vi "Read Single Raw Waveform.vi"(4 "Arm trigger":bool, 6 "Custom Source ID":string, 8 "error in (no error)":errorcluster, 9 "Timeout (10000 ms)":u32=10000, 10 "Source (0: Channel 1)":u16(ring) items=["Channel 1", "Channel 2", "Channel 3", "Channel 4", "Memory 1", "Memory 2", "Memory 3", "Memory 4", "Function 1", "Function 2", "Function 3", "Function 4", "Function 5", "Function 6", "Function 7", "Function 8", "Other"], 11 "VISA resource name":refnum<visa-resource-name>) -> (0 "error out":errorcluster, 2 "Waveform Data":waveform(i16)(graph), 3 "VISA resource name out":refnum<visa-resource-name>, 5 "Vertical offset":sgl, 7 "Vertical gain":sgl)   [LabVIEW 2018, in "LeCroy Wave Series.lvlib"]
doc: "Initiates an acquisition on all channels that you enabled with the <B>Configure Channel</B> VI. The VI waits for the acquisition to complete and returns the waveform for the Source channel you specified. If the oscilloscope did not complete the acquisition within the time period you specify with the Timeout parameter, the VI returns a time out error. A common cause for a timeout error is the acquisition was not triggered. For example, the trigger level is out of range of the waveform.\n\nCall the <B>Fetch Waveform</B> VI to obtain the waveforms for each of the remaining enabled Source channels without initiating another acquisition.\n\nNote: If your instrument does not support auto compensation for probe attenuation, you may need to adjust the scaling of the Waveform Data accordingly. This is handled automatically in the <B>Configure Channel</B> VI or can be done manually by multiplying the Waveform Data by the probe attenuation."
uses:
  LeCroy Wave Series.lvlib
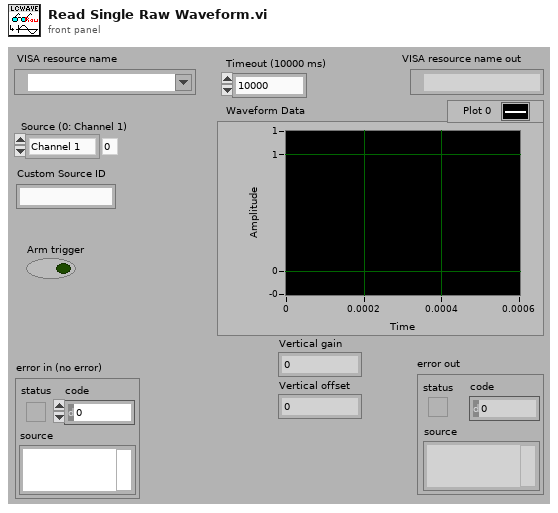
[diagram p1: front panel]
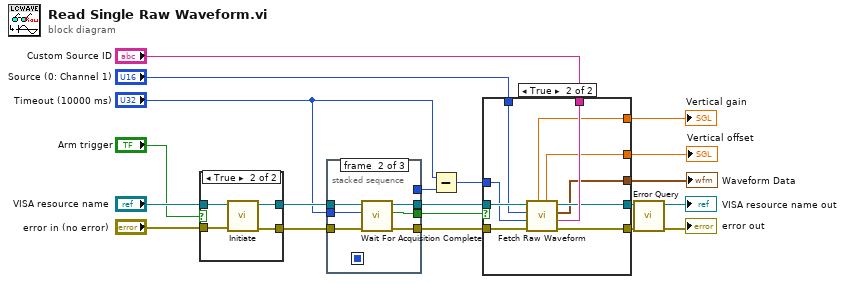
[diagram p0: block diagram]
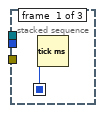
[diagram p4: hidden frame]
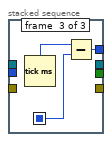
[diagram p5: hidden frame]
diagram:
  n1 = case shown="True" "Arm trigger" {
    tunnel: "VISA resource name" -> [w22 w26]
    tunnel: "error in (no error)" -> [w21 w25]
    tunnel: [w22 w24] -> w12
    tunnel: [w21 w23] -> w11
    frame False {
    }
    frame True {
      n2 = call "Initiate.vi"("error in (no error)"=w25, "VISA resource name"=w26) -> ("error out"=w23:errorcluster, "VISA resource name out"=w24:refnum<visa-resource-name>)  [unwired: 8 in]
    }
  }
  n3 = stacked-sequence {
    seq-local: [w27 _ _] -> [_ _ w35]
    tunnel: "Timeout (10000 ms)" -> [_ w33 _]
    tunnel: w12 -> [_ w31 _]
    tunnel: w11 -> [_ w29 _]
    tunnel: [_ w28 _] -> w10
    tunnel: [_ w30 _] -> w6
    tunnel: [_ _ w34] -> w8
    tunnel: [_ w32 _] -> w5
    frame #0 {
      n4 = Tick Count (ms)() -> (millisecond timer value=w27:u32)
    }
    frame #1 {
      n5 = call "Wait For Acquisition Complete.vi"("error in (no error)"=w29, "Timeout (10000 ms)"=w33, "VISA resource name"=w31) -> ("error out"=w28:errorcluster, "Complete"=w32:bool, "VISA resource name out"=w30:refnum<visa-resource-name>)  [unwired: 6 in]
    }
    frame #2 {
      n6 = Tick Count (ms)() -> (millisecond timer value=w36:u32)
      n7 = Subtract(x=w36, y=w35) -> (x-y=w34:u32)
    }
  }
  n8 = Subtract(x="Timeout (10000 ms)", y=w8) -> (x-y=w7:u32)
  n9 = case shown="True" w5 {
    tunnel: [_ w41] -> w18
    tunnel: [w38 w43] -> w17
    tunnel: [w37 w42] -> w15
    tunnel: "Source (0: Channel 1)" -> [_ w46]
    tunnel: w10 -> [w37 w47]
    tunnel: w7 -> [_ w45]
    tunnel: w6 -> [w38 w48]
    tunnel: "Custom Source ID" -> [_ w44]
    tunnel: [_ w40] -> w3
    tunnel: [_ w39] -> w2
    frame False {
    }
    frame True {
      n10 = call "Fetch Raw Waveform.vi"("Custom Source ID"=w44, "error in (no error)"=w47, "Timeout (10000 ms)"=w45, "Source (0: Channel 1)"=w46, "VISA resource name"=w48) -> ("error out"=w42:errorcluster, "Waveform Graph"=w41:waveform(i16), "VISA resource name out"=w43:refnum<visa-resource-name>, "Vertical offset"=w39:sgl, "Vertical gain"=w40:sgl)  [unwired: 2 in]
    }
  }
  "Waveform Data" <- w18
  "Vertical gain" <- w3
  "Vertical offset" <- w2
  n11 = call "Error Query.vi"("error in (no error)"=w15, "VISA resource name"=w17) -> ("error out"=→"error out":errorcluster, "VISA resource name out"=→"VISA resource name out":refnum<visa-resource-name>)  [unwired: 6 in, 2 out]
